vi "InitializeFpgaWithTachAcquisition.vi"(8 "error in (no error)":errorcluster, 11 "923x Acquisition Config":T1={"Acq"=FALSE, "NumberOfModules"=0, "Dynamic FPGA VI Ref"=refnum, "KeyphasorX3"=[], "FixedSizeX32"={"EnabledChannels"=[], "Sensitivity"=[], "InputConfig"=[]}, "SamplingInfo"={"Number of Channels"=4, "Sampling Rate"=4.0, "Channels"=[], "Units"=[], "Offsets"=[]}, "Normal Mode Sample Rate"=0.0, "BlockSize (sec)"=0.0, "Samples To Read (per chan)"=0, "RunningAcquisitionLength"=0.0, "Settling Time"=0.0, "Fpga Tach Buffer Size (samples)"=0, "Waveform Groups"=[], "Acquisition Block Number"=0, "Device Name"="", "ValidConfig"=FALSE, "Last Dynamic Module"="", "HighPassFilterState"=[], "Low Frequency Cutoff"=[], "BurstMode"={"Acquisition Time"=0.0, "Sample Rate"=0.0, "Collection Reason"=""}} {"HighPassFilterState"."Filter State" format="%.2f"; "HighPassFilterState"."IIR Filter Cluster"."Forward Coefficients" format="%.2f"; "HighPassFilterState"."IIR Filter Cluster"."Reverse Coefficients" format="%.2f"; "FixedSizeX32"."InputConfig" items=["AC Coupled", "DC Coupled", "IEPE AC Coupled"]}) -> (0 "error out":errorcluster, 1 "start acquisition?":bool, 2 "dynamic FPGA VI reference":refnum<k20>, 3 "923x Acquisition Config out":T1={"Acq"=FALSE, "NumberOfModules"=0, "Dynamic FPGA VI Ref"=refnum, "KeyphasorX3"=[], "FixedSizeX32"={"EnabledChannels"=[], "Sensitivity"=[], "InputConfig"=[]}, "SamplingInfo"={"Number of Channels"=4, "Sampling Rate"=4.0, "Channels"=[], "Units"=[], "Offsets"=[]}, "Normal Mode Sample Rate"=0.0, "BlockSize (sec)"=0.0, "Samples To Read (per chan)"=0, "RunningAcquisitionLength"=0.0, "Settling Time"=0.0, "Fpga Tach Buffer Size (samples)"=0, "Waveform Groups"=[], "Acquisition Block Number"=0, "Device Name"="", "ValidConfig"=FALSE, "Last Dynamic Module"="", "HighPassFilterState"=[], "Low Frequency Cutoff"=[], "BurstMode"={"Acquisition Time"=0.0, "Sample Rate"=0.0, "Collection Reason"=""}} {"HighPassFilterState"."Filter State" format="%.2f"; "HighPassFilterState"."IIR Filter Cluster"."Forward Coefficients" format="%.2f"; "HighPassFilterState"."IIR Filter Cluster"."Reverse Coefficients" format="%.2f"; "FixedSizeX32"."InputConfig" items=["AC Coupled", "DC Coupled", "IEPE AC Coupled"]})   [LabVIEW 2017, in "CmsAcquisition.lvlib"]
doc: "Initializes the acquisition of the dynamic channels with the RIO Wfm API."
uses:
  <vilib>/addons/InsightCM/Devices/Shared/Cms/CmsAcquisition/CmsAcquisition.lvlib
  <vilib>/addons/InsightCM/Devices/Shared/Cms/CmsAcquisition/controls/Configuration.ctl
  <vilib>/addons/InsightCM/Devices/Shared/Cms/CmsAcquisition/controls/TachometerConfig.ctl
  <vilib>/addons/InsightCM/Devices/Shared/Cms/CmsAcquisition/controls/FixedSizeArrays.ctl
  <vilib>/LabVIEW Targets/FPGA/cRIO/shared/nicrio_ModuleControls/nicrio_cRIO-9232_ConfigModeRing.ctl
  <vilib>/addons/InsightCM/Devices/Shared/Cms/cRIOWfmAcq/subVIs/RIO Wfm Cust Ctrls/rwfm_SamplingInfo.ctl
  <vilib>/addons/InsightCM/Devices/Shared/Cms/CmsAcquisition/controls/Group.ctl
  <vilib>/addons/InsightCM/Devices/Shared/Cms/CmsAcquisition/controls/Channel.ctl
  <vilib>/addons/InsightCM/Utilities/Analysis/Vibration/controls/HighPassFilterState.ctl
  <vilib>/addons/InsightCM/Devices/Shared/Cms/CmsAcquisition/controls/BurstMode.ctl
  <vilib>/Utility/error.llb/Error Cluster From Error Code.vi
  <vilib>/rvi/errors/niLvFpgaAdjustHostInterfaceError.vi
  <vilib>/rvi/interface/nirviReadWriteControl/nirviReadWriteControl.xnode
  <vilib>/addons/InsightCM/Devices/Shared/Cms/cRIOWfmAcq/subVIs/RIO Wfm Cust Ctrls/rwfm_FPGARefTach.ctl
  <vilib>/addons/InsightCM/Devices/Shared/Cms/cRIOWfmAcq/cRIOWfmLib.lvlib
  <vilib>/rvi/interface/Simulation/niFpgaSimulationCallBeginRW.vi
  NiFpgaLv.dll
  <vilib>/addons/InsightCM/Utilities/Analysis/Vibration/VibrationAnalysisFunctions.lvlib
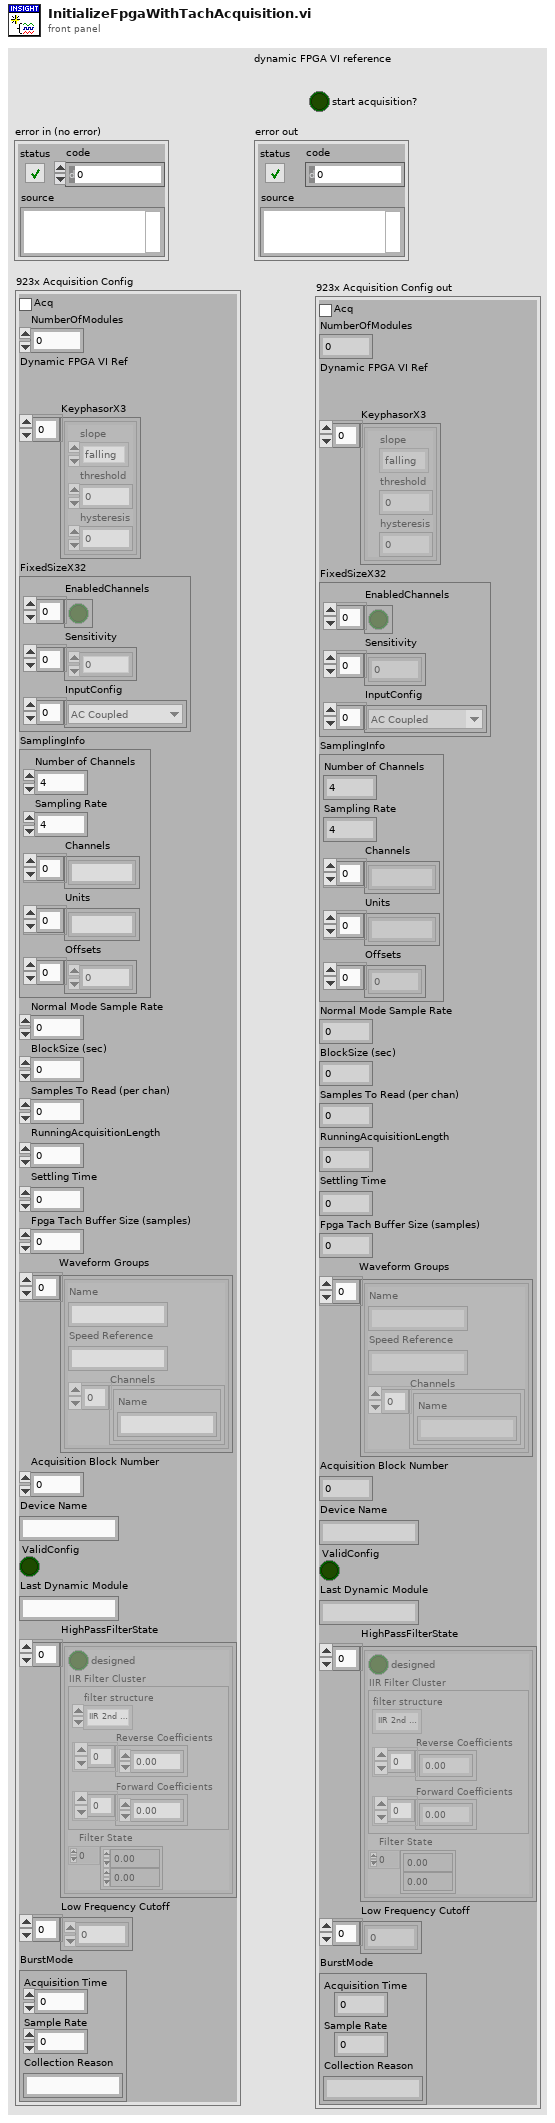
[diagram p1: front panel]
types:
  T1 = typedef "CmsAcquisition.lvlib/Configuration.ctl" = cluster{"Acq":bool, "NumberOfModules":i16, "Dynamic FPGA VI Ref":refnum<k20>, "KeyphasorX3":T2[], "FixedSizeX32":T3, "SamplingInfo":T5, "Normal Mode Sample Rate":dbl, "BlockSize (sec)":dbl, "Samples To Read (per chan)":i32, "RunningAcquisitionLength":dbl, "Settling Time":dbl, "Fpga Tach Buffer Size (samples)":i32, "Waveform Groups":T6[], "Acquisition Block Number":i32, "Device Name":string, "ValidConfig":bool, "Last Dynamic Module":string, "HighPassFilterState":T8[], "Low Frequency Cutoff":dbl[], "BurstMode":T9}
  T2 = typedef "CmsAcquisition.lvlib/TachometerConfig.ctl" = cluster{"slope":enum16{"falling", "rising"}, "threshold":dbl, "hysteresis":dbl}
  T3 = typedef "CmsAcquisition.lvlib/FixedSizeArrays.ctl" = cluster{"EnabledChannels":bool[], "Sensitivity":dbl[], "InputConfig":T4[]}
  T4 = typedef "nicrio_cRIO-9232_ConfigModeRing.ctl" = u8
  T5 = typedef "cRIOWfmLib.lvlib/rwfm_SamplingInfo.ctl" = cluster{"Number of Channels":i32, "Sampling Rate":dbl, "Channels":string[], "Units":string[], "Offsets":sgl[]}
  T6 = typedef "CmsAcquisition.lvlib/Group.ctl" = cluster{"Name":string, "Speed Reference":string, "Channels":T7[]}
  T7 = typedef "CmsAcquisition.lvlib/Channel.ctl" = cluster{"Name":string}
  T8 = typedef "VibrationAnalysisFunctions.lvlib/HighPassFilterState.ctl" = cluster{"designed":bool, "IIR Filter Cluster":cluster{"filter structure":enum32{"IIR 2nd Order", "IIR 4th Order"}, "Reverse Coefficients":dbl[], "Forward Coefficients":dbl[]}, "Filter State":dbl[]}
  T9 = typedef "CmsAcquisition.lvlib/BurstMode.ctl" = cluster{"Acquisition Time":dbl, "Sample Rate":dbl, "Collection Reason":string}
  T10 = typedef "cRIOWfmLib.lvlib/rwfm_FPGARefTach.ctl" = refnum<k20>
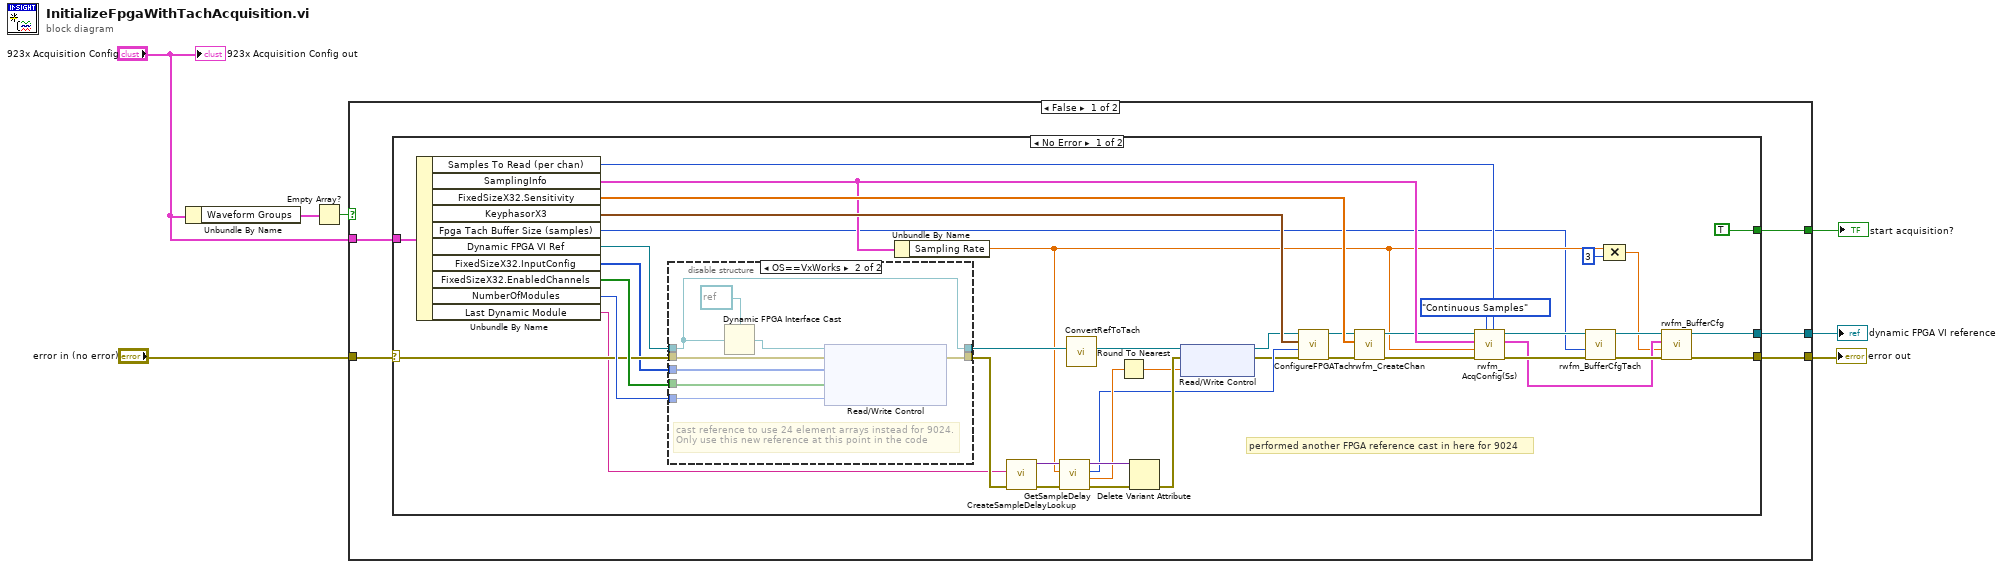
[diagram p0: block diagram]
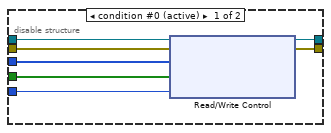
[diagram p2: hidden frame]
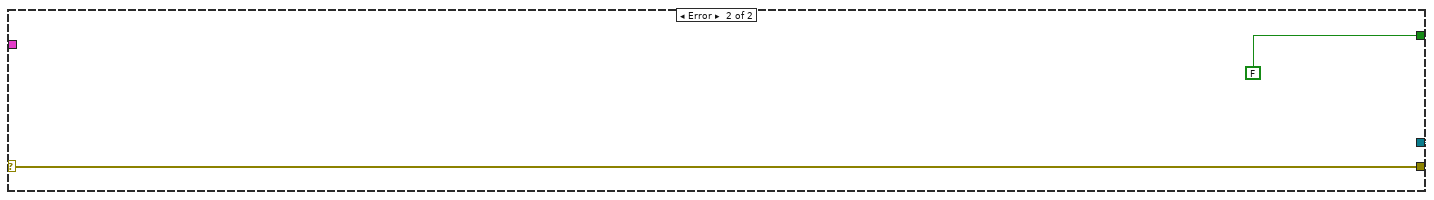
[diagram p3: hidden frame]
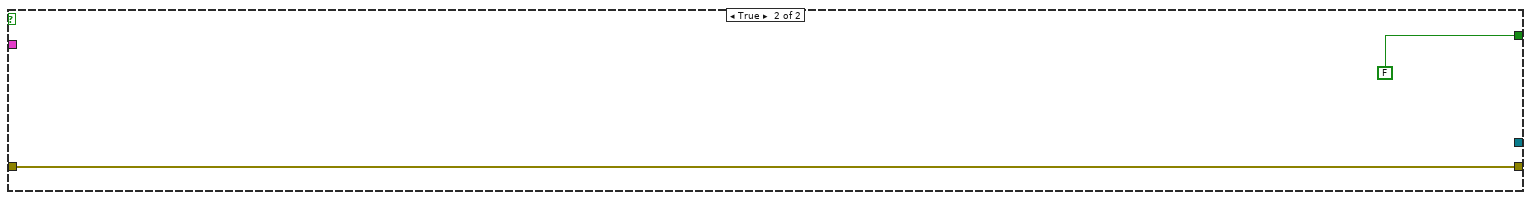
[diagram p4: hidden frame]
diagram:
  n1 = Unbundle By Name("923x Acquisition Config") -> ("Waveform Groups"=w3:T6[])
  n2 = Empty Array?(array=w3) -> (empty?=w2:bool)
  n3 = case shown="False" w2 {
    tunnel: [w12 w73] -> w7
    tunnel: "error in (no error)" -> [w11 w73]
    tunnel: [w10 _] -> w5
    tunnel: "923x Acquisition Config" -> [w9 _]
    tunnel: [w8 FALSE] -> w1
    frame False {
      n4 = case shown="No Error" w11 {
        selector: w11 -> [w28 w71]
        tunnel: w9 -> [w51 _]
        tunnel: [w50 w71] -> w12
        tunnel: [w49 refnum<k0> refnum] -> w10
        tunnel: [TRUE FALSE] -> w8
        frame No Error {
          # "performed another FPGA reference cast in here for 9024"
          n5 = Unbundle By Name(w51) -> ("Samples To Read (per chan)"=w45:i32, "SamplingInfo"=w47:T5, "FixedSizeX32.Sensitivity"=w52:dbl[], "KeyphasorX3"=w48:T2[], "Fpga Tach Buffer Size (samples)"=w13:i32, "Dynamic FPGA VI Ref"=w14:refnum<k20>, "FixedSizeX32.InputConfig"=w20:T4[], "FixedSizeX32.EnabledChannels"=w53:bool[], "NumberOfModules"=w46:i16, "Last Dynamic Module"=w15:string)
          n6 = disable-structure shown="OS==VxWorks" {
            disable-tunnel: w53 -> [w60 w62]
            disable-tunnel: w46 -> [w59 w68]
            disable-tunnel: [w58 w67] -> w37
            disable-tunnel: w28 -> [w57 w66]
            disable-tunnel: [w56 w61] -> w27
            disable-tunnel: w20 -> [w55 w63]
            disable-tunnel: w14 -> [w54 w61]
            frame condition #0 (active) {
              n7 = xnode "Read/Write Control"("FPGA VI Reference In"=w54, "error in"=w57, "Input Config Array"=w55, "Enable Chan Array"=w60, "Number of Modules"=w59) -> ("FPGA VI Reference Out"=w56:refnum<k20>, "error out"=w58:errorcluster)
            }
            frame condition #1 {
              # "cast reference to use 24 element arrays instead for 9024.\nOnly use this new reference at this point in the code"
              n8 = Dynamic FPGA Interface Cast(Session In=refnum<k20> refnum ("FPGA VI Reference In"), Type=w61) -> (Session Out=w64:refnum<k20>)
              n9 = xnode "Read/Write Control"("FPGA VI Reference In"=w64, "error in"=w66, "Input Config Array"=w63, "Enable Chan Array"=w62, "Number of Modules"=w68) -> ("error out"=w67:errorcluster)  [unwired: 1 out]
            }
          }
          n10 = Unbundle By Name(w47) -> ("Sampling Rate"=w18:dbl)
          n11 = call <vilib>:"CreateSampleDelayLookup.vi"("error in"=w37, "Last Dynamic Module"=w15) -> ("error out"=w38:errorcluster, "lookup"=w41:variant)  [unwired: 8 in]
          n12 = call <vilib>:"GetSampleDelay.vi"("error in (no error)"=w38, "sample rate"=w18, "lookup"=w41) -> ("error out"=w40:errorcluster, "delay compensation (samples)"=w32:dbl, "delay compensation (OS clocks)"=w30:u32, "lookup"=w39:variant)  [unwired: 5 in]
          n13 = call <vilib>:"ConvertRefToTach.vi"("FPGA Ref"=w27) -> ("FPGA Ref"=w26:T10)  [unwired: 10 in]
          n14 = Round To Nearest(number=w32) -> (nearest integer value=w29:dbl)
          n15 = Delete Variant Attribute(4:w40, 7:w39) -> (0:w31:errorcluster)  [unwired: 1 in, 2 out]
          n16 = xnode "Read/Write Control"("FPGA VI Reference In"=w26, "error in"=w31, "Tach Delay"=w29) -> ("FPGA VI Reference Out"=w21:T10, "error out"=w25:errorcluster)
          n17 = call <vilib>:"ConfigureFPGATach.vi"("error in (no error)"=w25, "delay comp"=w30, "keyphasor config"=w48, "dynamic FPGA VI reference"=w21) -> ("error out"=w42:errorcluster, "dynamic FPGA VI reference"=w23:T10)  [unwired: 6 in]
          n18 = call <vilib>:"rwfm_CreateChan.vi"("error in"=w42, "Sensitivity"=w52, "Dynamic FPGA VI Reference"=w23) -> ("error out"=w43:errorcluster, "Dynamic FPGA VI Reference"=w24:T10)  [unwired: 7 in]
          n19 = call <vilib>:"rwfm_AcqConfig(Ss).vi"("Samples per Channel"=w45, "Sample Mode"=enum16{"Finite Samples", "Continuous Samples"}."Continuous Samples", "error in"=w43, "Sample Rate S/s"=w18, "Sampling Info In"=w47, "Dynamic FPGA Ref"=w24) -> ("error out"=w34:errorcluster, "Sampling Info Out"=w33:T5, "Dynamic FPGA Ref Out"=w22:T10)  [unwired: 2 in, 1 out]
          n20 = call <vilib>:"rwfm_BufferCfgTach.vi"("error in"=w34, "Buffer Size [Total Samples]"=w13, "Dynamic FPGA VI Reference"=w22) -> ("error out"=w35:errorcluster, "FPGA VI Reference Out"=w36:T10)  [unwired: 6 in, 1 out]
          n21 = Compound Arithmetic op=MULTIPLY(w18, 3 ("value")) -> (w17:dbl)
          n22 = call <vilib>:"rwfm_BufferCfg.vi"("error in"=w35, "Buffer Size [Samps per Chan]"=w17, "Sampling Info In"=w33, "Dynamic FPGA VI Reference"=w36) -> ("error out"=w50:errorcluster, "Dynamic FPGA VI Reference"=w49:T10)  [unwired: 4 in, 2 out]
        }
        frame Error {
        }
      }
    }
    frame True {
    }
  }
  "error out" <- w7
  "dynamic FPGA VI reference" <- w5
  "start acquisition?" <- w1
  "923x Acquisition Config out" <- "923x Acquisition Config"
